vi "Control to Key List.vi"(5 "section":string, 7 "Prefix":string, 8 "Error In":errorcluster, 11 "Ctl Refnum":refnum<vi>) -> (0 "Error Out":errorcluster, 3 "Ctl Refnum out":refnum<vi>)   [LabVIEW 2015]
uses:
  <vilib>/Utility/Data Type/NI_Data Type.lvlib
panel:
  out "Key list":T1
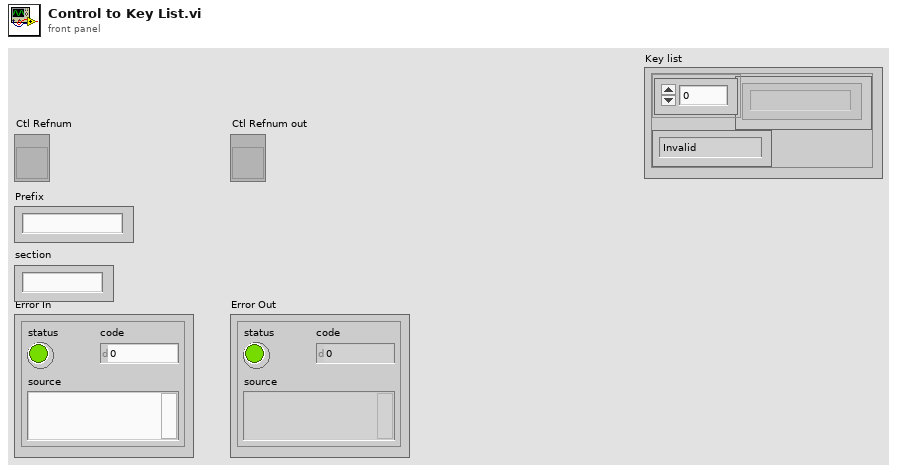
[diagram p1: front panel]
types:
  T1 = cluster{"Array":string[], "Enum":enum16{"Invalid", "Boolean", "Double", "I32", "Path", "String", "U32", "Array", "Cluster"}}
  T2 = typedef "NI_Data Type.lvlib/Data Type.ctl" = enum8{"Invalid Type", "Void", "I8", "I16", "I32", "I64", "U8", "U16", "U32", "U64", "Single Float", "Double Float", "Extended Float", "Single Complex", "Double Complex", "Extended Complex", "Enum U8", "Enum U16", "Enum U32", "Enum U64", "Single Float With Unit", "Double Float With Unit", "Extended Float With Unit", "Single Complex with Unit", "Double Complex with Unit", "Extended Complex with Unit", "Boolean", "String", "Path", "Picture", "Tag", "Array", "Cluster", "Variant", "LV Variant", "Waveform", "Timestamp", "Digital Waveform", "Digital Data", "ExpressData", "Refnum", "External Data", "VI", "Poly VI", "LabVIEW Class Instance", "Fixed Point"}
  T3 = enum16{"Invalid", "Boolean", "Double", "I32", "Path", "String", "U32", "Array", "Cluster"}
  T4 = cluster{string[], enum16{"Invalid", "Boolean", "Double", "I32", "Path", "String", "U32", "Array", "Cluster"}}
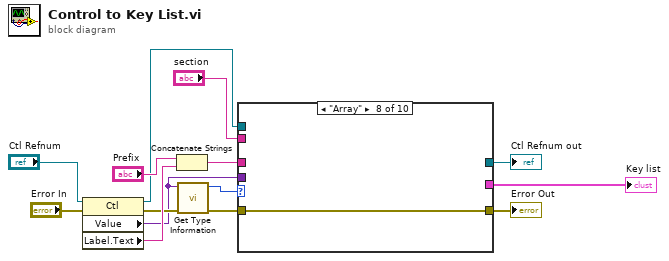
[diagram p0: block diagram]
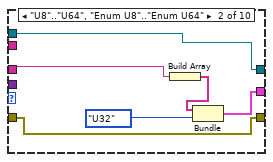
[diagram p3: hidden frame]
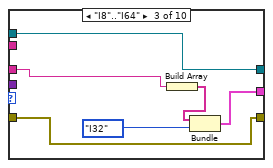
[diagram p4: hidden frame]
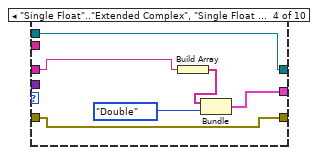
[diagram p5: hidden frame]
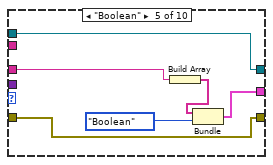
[diagram p6: hidden frame]
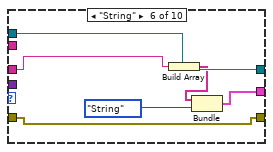
[diagram p7: hidden frame]
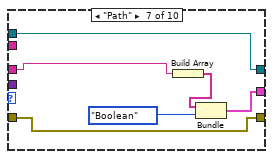
[diagram p8: hidden frame]
diagram:
  n1 = property class="Ctl"(reference="Ctl Refnum", error in="Error In") -> (reference out=w8:refnum<vi>, error out=w7:errorcluster, "Value"=w2:variant, "Label.Text"=w11:string)
  n2 = Concatenate Strings("Prefix", w11) -> (w9:string)
  n3 = call <vilib>:"Get Type Information.vi"("error in (no error)"=w7, "Variant"=w2) -> ("error out"=w6:errorcluster, "Type"=w13:T2)  [unwired: 5 in, 3 out]
  n4 = case shown="\"Array\"" w13 {
    tunnel: "section" -> [_ _ _ _ _ _ _ _ _ _]
    tunnel: w9 -> [_ w19 w23 w30 w40 w42 w47 _ _ _]
    tunnel: w8 -> [w15 w22 w28 w29 w36 w46 w48 _ _ _]
    tunnel: w6 -> [w16 w17 w25 w32 w37 w43 w50 w53 _ _]
    tunnel: [w15 w22 w28 w29 w36 w46 w48 _ _ _] -> w5
    tunnel: [w16 w17 w25 w32 w37 w43 w50 w53 _ _] -> w4
    tunnel: w2 -> [_ _ _ _ _ _ _ _ _ _]
    tunnel: [_ w18 w24 w31 w35 w41 w49 _ _ _] -> w1
    frame "Invalid Type", Default {
    }
    frame "U8".."U64", "Enum U8".."Enum U64" {
      n5 = Build Array(w19) -> (w21:string[])
      n6 = Bundle(w21, T3."U32") -> (w18:T4)  [unwired: 1 in]
    }
    frame "I8".."I64" {
      n7 = Build Array(w23) -> (w27:string[])
      n8 = Bundle(w27, T3."I32") -> (w24:T4)  [unwired: 1 in]
    }
    frame "Single Float".."Extended Complex", "Single Float With Unit".."Extended Complex with Unit" {
      n9 = Build Array(w30) -> (w34:string[])
      n10 = Bundle(w34, T3."Double") -> (w31:T4)  [unwired: 1 in]
    }
    frame "Boolean" {
      n11 = Build Array(w40) -> (w39:string[])
      n12 = Bundle(w39, T3."Boolean") -> (w35:T4)  [unwired: 1 in]
    }
    frame "String" {
      n13 = Build Array(w42) -> (w45:string[])
      n14 = Bundle(w45, T3."String") -> (w41:T4)  [unwired: 1 in]
    }
    frame "Path" {
      n15 = Build Array(w47) -> (w52:string[])
      n16 = Bundle(w52, T3."Boolean") -> (w49:T4)  [unwired: 1 in]
    }
    frame "Array" {
    }
    frame "Cluster" {
    }
    frame "Fixed Point" {
    }
  }
  "Ctl Refnum out" <- w5
  "Error Out" <- w4
  "Key list" <- w1
